vi "Get File Path.vi"(8 "error in (no error)":errorcluster, 11 "Handler.File in":refnum<class "Handler.File.lvclass">) -> (0 "error out":errorcluster, 2 "File Path":path, 3 "Handler.File out":refnum<class "Handler.File.lvclass">)   [LabVIEW 2017, in "Error Log.lvlib" / "Handler.File.lvclass"]
uses:
  Handler.File.lvclass
  Handler.File.lvclass/Handler.File.ctl
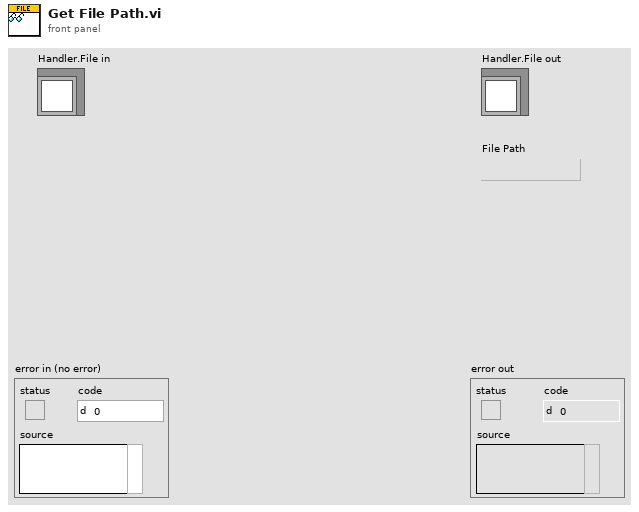
[diagram p1: front panel]
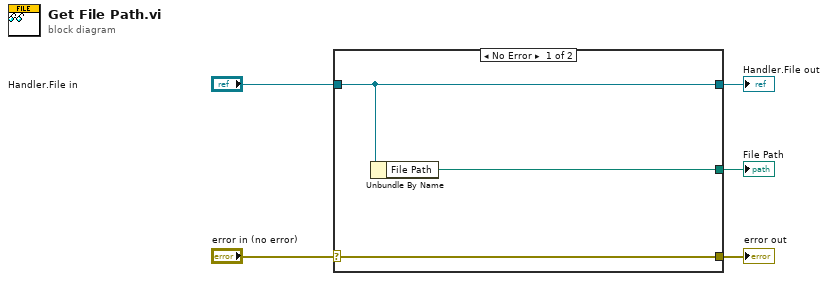
[diagram p0: block diagram]
diagram:
  n1 = case shown="No Error" "error in (no error)" {
    selector: "error in (no error)" -> [w8 w9]
    tunnel: [w8 w9] -> w4
    tunnel: [w7 w10] -> w2
    tunnel: "Handler.File in" -> [w7 w10]
    tunnel: [w6 _] -> w1
    frame No Error {
      n2 = Unbundle By Name(w7) -> ("File Path"=w6:path)
    }
    frame Error {
    }
  }
  "error out" <- w4
  "Handler.File out" <- w2
  "File Path" <- w1
